vi "异常处理_1.vi"(10 "file path (use dialog)":path) -> (1 "error constant":errorcluster, 2 "String":string)   [LabVIEW 2023]
panel:
  # "错误处理"
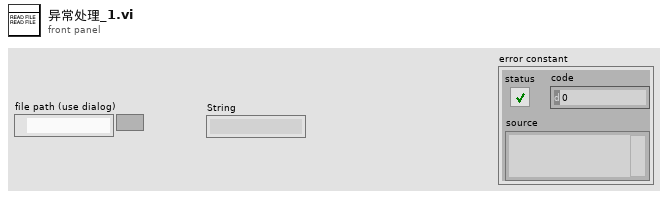
[diagram p1: front panel]
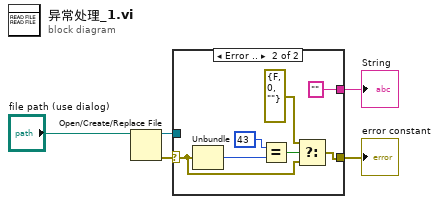
[diagram p0: block diagram]
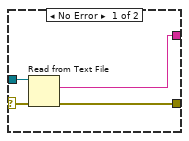
[diagram p2: hidden frame]
diagram:
  n1 = Open/Create/Replace File(file path (use dialog)="file path (use dialog)") -> (refnum out=w5:refnum<file>, error out=w4:errorcluster)  [unwired: 5 in, 1 out]
  n2 = case shown="Error .." w4 {
    selector: w4 -> [w8 w10]
    tunnel: w5 -> [w9 _]
    tunnel: [w7 w12] -> w2
    tunnel: [w6 ""] -> w3
    frame No Error {
      n3 = Read from Text File(file (use dialog)=w9, error in=w8) -> (text=w6:string, error out=w7:errorcluster)  [unwired: 2 in, 2 out]
    }
    frame Error {
      n4 = Unbundle(w10) -> ("code"=w16:i32)  [unwired: 2 out]
      n5 = Equal?(x=43, y=w16) -> (x = y?=w14:bool)
      n6 = Select(t=errorcluster {"status"=FALSE, "code"=0, "source"=""} ("error constant"), s=w14, f=w10) -> (s? t:f=w12:errorcluster)
    }
  }
  "String" <- w3
  "error constant" <- w2
